vi "Basic 1.vi"() -> ()   [LabVIEW 2014, in "Arduino TFT.lvlib"]
uses:
  <vilib>/Aledyne-TSXperts/Arduino Compatible Compiler for LabVIEW/addons/Arduino TFT/Arduino TFT.lvlib
  <vilib>/Aledyne-TSXperts/Arduino Compatible Compiler for LabVIEW/Arduino Compatible Compiler for LabVIEW.lvlib
panel:
  out "Error Out":errorcluster
  in  "Error In":errorcluster
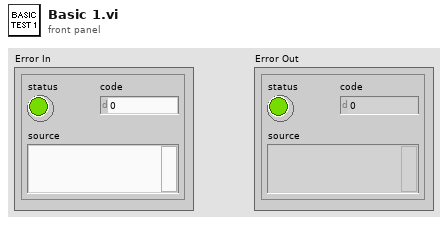
[diagram p1: front panel]
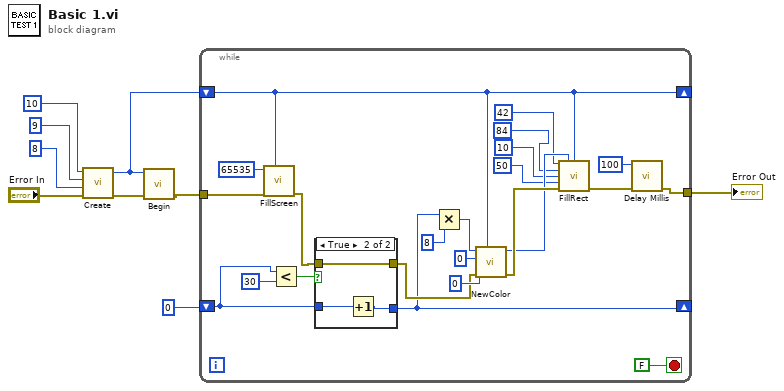
[diagram p0: block diagram]
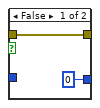
[diagram p2: hidden frame]
diagram:
  n1 = call <vilib>:"Create.vi"("Error In"="Error In", "rst"=u8 8 ("cs"), "rs"=u8 9 ("cs"), "cs"=u8 10) -> ("Error Out"=w5:errorcluster, "Instance"=w3:u32)  [unwired: 4 in]
  n2 = call <vilib>:"Begin.vi"("Error In"=w5, "Instance"=w3) -> ("Error Out"=w4:errorcluster)  [unwired: 8 in]
  n3 = while {
    tunnel: w4 -> [w31]
    tunnel: [w21] -> w2
    shift-right: [w10] -> _
    shift-left: w3 -> [w10]
    shift-right: [w13] -> _
    shift-left: u8 0 ("green") -> [w17]
    stop <- FALSE stop-if-true
    n4 = call <vilib>:"FillScreen.vi"("Instance"=w10, "Error In"=w31, "color"=u16 65535) -> ("Error Out"=w16:errorcluster)  [unwired: 8 in]
    n5 = Less?(x=w17, y=u8 30) -> (x < y?=w19:bool)
    n6 = case shown="True" w19 {
      tunnel: w17 -> [_ w37]
      tunnel: [u8 0 w36] -> w13
      tunnel: w16 -> [w33 w35]
      tunnel: [w33 w35] -> w15
      frame False {
      }
      frame True {
        n7 = Increment(x=w37) -> (x+1=w36:u8)
      }
    }
    n8 = Multiply(x=w13, y=u8 8 ("green")) -> (x*y=w12:u8)
    n9 = call <vilib>:"NewColor.vi"("Instance"=w10, "Error In"=w15, "blue"=u8 0, "green"=u8 0, "red"=w12) -> ("Error Out"=w28:errorcluster, "color"=w27:u16)  [unwired: 5 in]
    n10 = call <vilib>:"FillRect.vi"("x"=u8 42, "color"=w27, "Instance"=w10, "y"=u8 84 ("x"), "width"=u8 10 ("x"), "height"=u8 50 ("x"), "Error In"=w28) -> ("Error Out"=w22:errorcluster)  [unwired: 8 in]
    n11 = call <vilib>:"Delay Millis.vi"("error in (no error)"=w22, "delay"=u32 100) -> ("error out"=w21:errorcluster)  [unwired: 9 in]
  }
  "Error Out" <- w2
